vi "SEN_Loop.vi"() -> ()   [LabVIEW 2020, in "GameController_SEN.lvlib"]
uses:
  GameController_SEN.lvlib
  Shared Code/TypeDefs/Cluster_Controller Buzz.ctl
  ENUM_SEN_State.ctl
  Shared Code/TypeDefs/ENUM_Controller Buzz Select.ctl
  <vilib>/Rock Robotics/WPI/Joystick/WPI_JoystickDevRef.ctl
  <vilib>/Rock Robotics/WPI/Joystick/WPI_JoystickDeviceEnum.ctl
  ENUM_SEN_Action.ctl
  6bb8d52f-ddc5-4686-9cd9-70e339759792.vi
  bc1d27d1-f877-4a00-a1ce-faa161c31405.vi
  Utility/Global_STOP.vi
  Global_CMD_Data In.vi
  Global_SEN_Data Out.vi
panel:
  out "State":T1
  in  "Tab Control":enum32{"NONE", "Test"}(tab)
  in  "BUZZ Select":T2
  in  "BUZZ Number":dbl min=0.0 max=1.0 step=0.1 format="%.1f"
  in  "Controller BUZZ":T3
  out "Input Bool Data":bool
  out "Output DBL Data":dbl
  out "Cycle Time (S)":dbl format="%.3g"
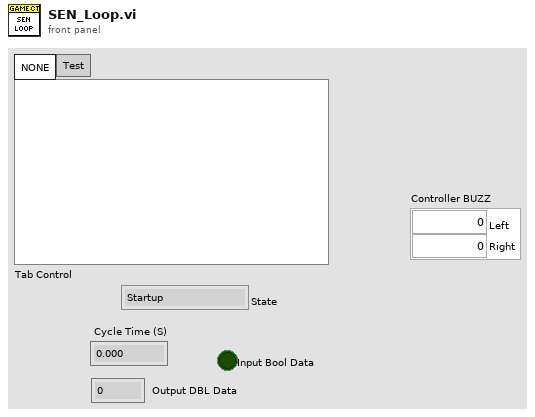
[diagram p1: front panel]
types:
  T1 = typedef "GameController_SEN.lvlib/ENUM_SEN_State.ctl" = enum16{"Startup", "Waiting BUZZ ON", "Shutdown", "Buzzing FULL Timed", "Waiting BUZZ OFF", "Buzzing Cycle Count", "Buzzing Intensity"}
  T2 = typedef "ENUM_Controller Buzz Select.ctl" = enum16{"None", "Timed Full ON", "Set Intensity", ".5 Sec Cycle Count"}
  T3 = typedef "Cluster_Controller Buzz.ctl" = cluster{"Left":dbl, "Right":dbl}
  T4 = typedef "WPI_JoystickDevRef.ctl" = cluster{"Device":T5}
  T5 = typedef "WPI_JoystickDeviceEnum.ctl" = enum16{"USB 0", "USB 1", "USB 2", "USB 3", "USB 4", "USB 5"}
  T6 = cluster{"Sensor Ref 1":T4, "Sensor Ref 0":T4, "State":T1, "Previous State":T1, "Current Time":timestamp, "Previous Time":timestamp, "Start Time":timestamp, "Target Time (ms)":u32, "Cycle Time(S)":dbl, "SEN Input":bool, "SEN Output DBL":dbl, "Read Enable":bool, "Axes 0":dbl[], "Buttons 0":bool[], "POVs 0":i16[], "Axes 1":dbl[], "Buttons 1":bool[], "POVs 1":i16[], "Controller BUZZ":T3, "BUZZ Select":T2, "BUZZ Number":dbl, "Target Number":dbl, "Count":i32, "BUZZ Target":T2}
  T7 = enum16{"Done", "First Call", "First Check", "BUZZ Match"}
  T8 = enum16{"Done", "First Call", "First Check", "BUZZ Match", "Time Expired", "Cycle Complete"}
  T9 = typedef "GameController_SEN.lvlib/ENUM_SEN_Action.ctl" = enum16{"No Action", "Reset Time", "Read Enable", "Read Disable", "SET Buzz"}
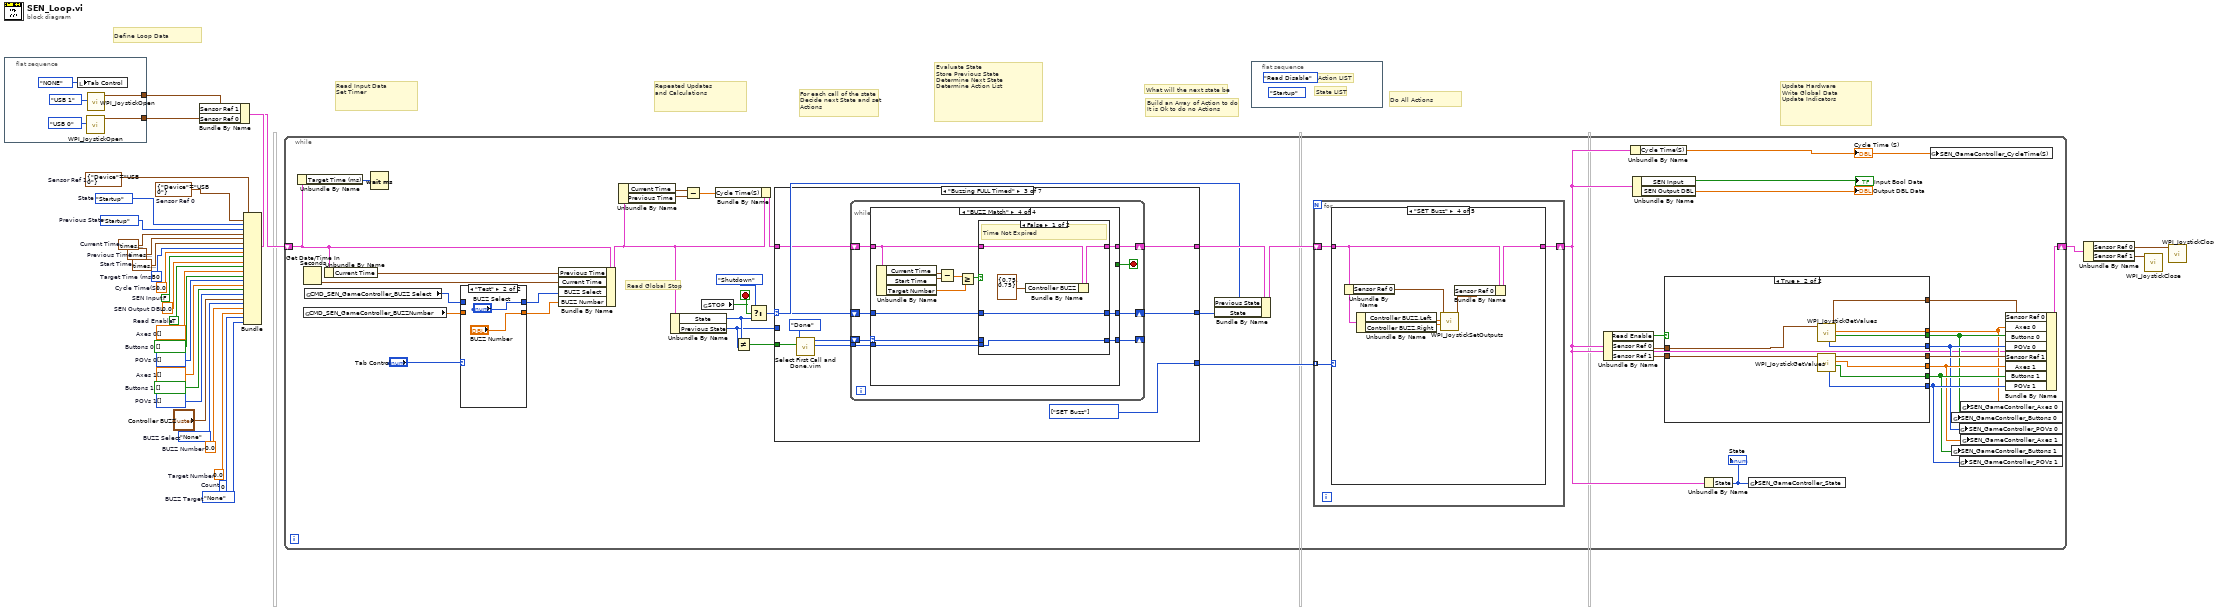
[diagram p0: block diagram]
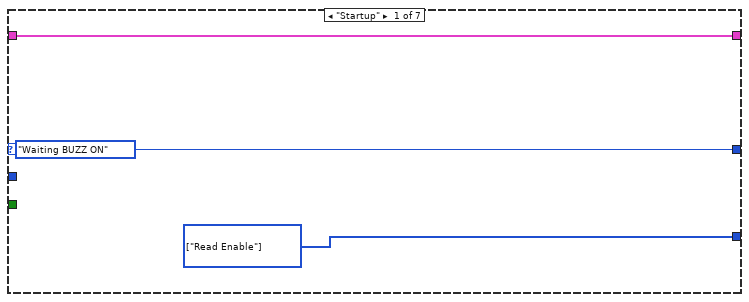
[diagram p3: hidden frame]
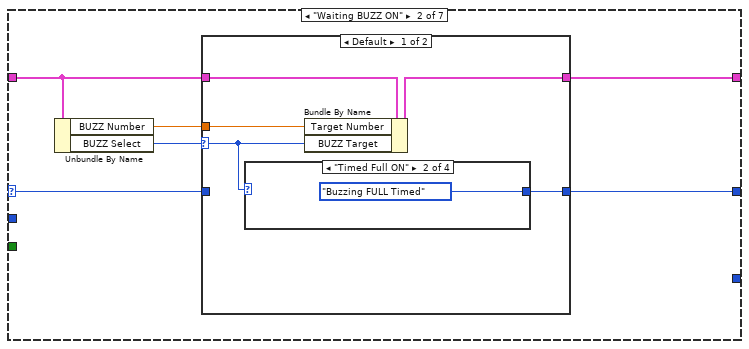
[diagram p4: hidden frame]
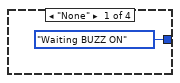
[diagram p5: hidden frame]
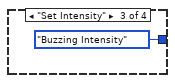
[diagram p6: hidden frame]
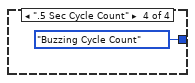
[diagram p7: hidden frame]
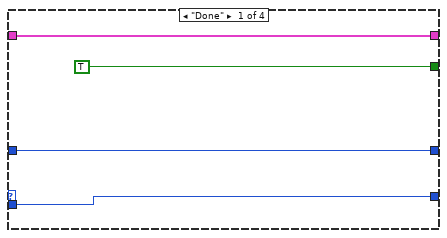
[diagram p9: hidden frame]
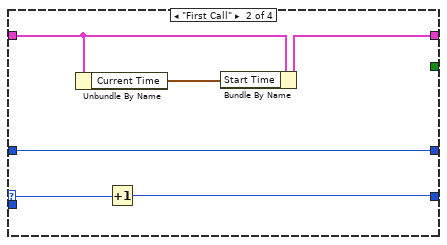
[diagram p10: hidden frame]
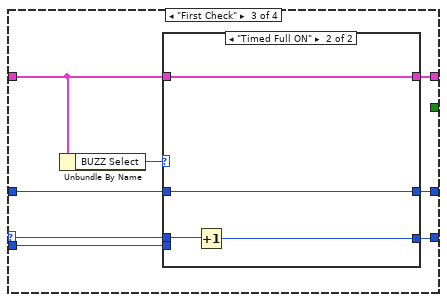
[diagram p11: hidden frame]
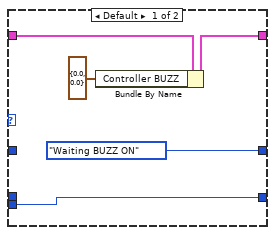
[diagram p12: hidden frame]
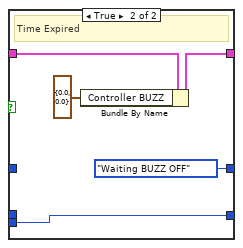
[diagram p13: hidden frame]
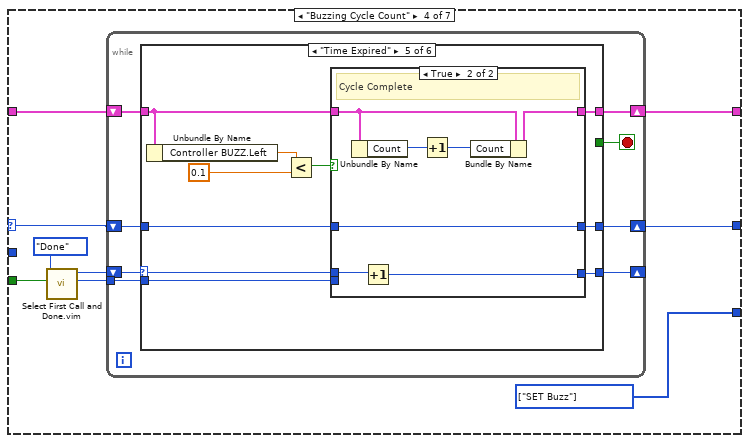
[diagram p14: hidden frame]
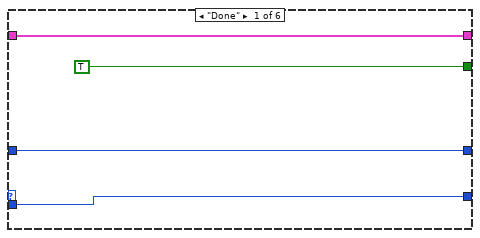
[diagram p15: hidden frame]
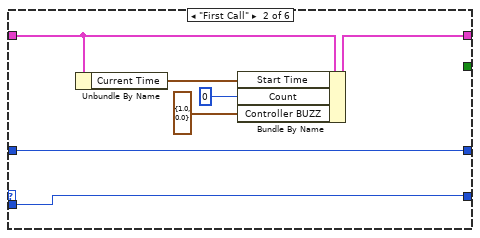
[diagram p16: hidden frame]
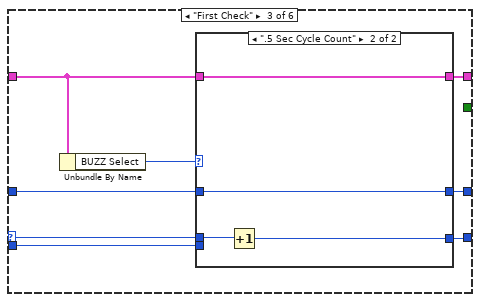
[diagram p17: hidden frame]
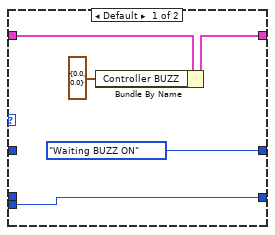
[diagram p18: hidden frame]
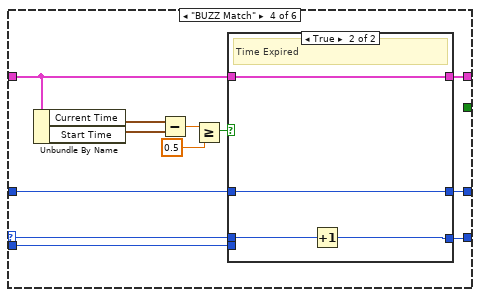
[diagram p19: hidden frame]
diagram:
  w1 = ENUM_Controller_Buzz_Select."None"  # BUZZ Target
  w2 = 0  # Count
  w3 = 0.0  # Target Number
  w4 = 0.0  # BUZZ Number
  w5 = ENUM_Controller_Buzz_Select."None"  # BUZZ Select
  w7 = T4 {"Device"=enum."USB 0"}  # Sensor Ref 0
  w8 = T4 {"Device"=enum."USB 0"}  # Sensor Ref 1
  w11 = i16[] []  # POVs 1
  w12 = bool[] []  # Buttons 1
  w13 = dbl[] []  # Axes 1
  w14 = i16[] []  # POVs 0
  w15 = bool[] []  # Buttons 0
  w16 = dbl[] []  # Axes 0
  w21 = TRUE  # Read Enable
  w23 = 0.0  # Cycle Time(S)
  w24 = ENUM_SEN_State."Startup"  # Previous State
  w25 = timestamp(0 s since 1904-01-01)  # Previous Time
  w26 = u32 50  # Target Time (ms)
  w27 = 0.0  # SEN Output DBL
  w28 = FALSE  # SEN Input
  w29 = timestamp(0 s since 1904-01-01)  # Start Time
  w30 = timestamp(0 s since 1904-01-01)  # Current Time
  w31 = ENUM_SEN_State."Startup"  # State
  # "Build an Array of Action to do\nIt is Ok to do no Actions"
  # "What will the next state be"
  # "For each call of the state\nDecide next State and set\nActions"
  # "Define Loop Data"
  # "Repeated Updates\nand Calculations"
  # "Read Input Data\nSet Timer"
  # "Evaluate State\nStore Previous State\nDetermine Next State\nDetermine Action List"
  # "Do All Actions"
  # "Update Hardware\nWrite Global Data\nUpdate Indicators"
  n1 = flat-sequence {
    tunnel: [w35] -> w18
    tunnel: [w33] -> w17
    frame #0 {
      n2 = local write "Tab Control"(enum32{"NONE", "Test"}."NONE" ("Tab Control")) -> ()
      n3 = call <vilib>:"WPI_JoystickOpen.vi"("JoystickDevice"=WPI_JoystickDeviceEnum."USB 0") -> ("JoystickDevRef"=w35:T4)  [unwired: 10 in]
      n4 = call <vilib>:"WPI_JoystickOpen.vi"("JoystickDevice"=WPI_JoystickDeviceEnum."USB 1") -> ("JoystickDevRef"=w33:T4)  [unwired: 10 in]
    }
  }
  n5 = Bundle("Sensor Ref 1"=w8, "Sensor Ref 0"=w7, "State"=w31, "Previous State"=w24, "Current Time"=w30, "Previous Time"=w25, "Start Time"=w29, "Target Time (ms)"=w26, "Cycle Time(S)"=w23, "SEN Input"=w28, "SEN Output DBL"=w27, "Read Enable"=w21, "Axes 0"=w16, "Buttons 0"=w15, "POVs 0"=w14, "Axes 1"=w13, "Buttons 1"=w12, "POVs 1"=w11, "Controller BUZZ"="Controller BUZZ", "BUZZ Select"=w5, "BUZZ Number"=w4, "Target Number"=w3, "Count"=w2, "BUZZ Target"=w1) -> (w20:T6)  [unwired: 1 in]
  n6 = Bundle By Name(cluster=w20, "Sensor Ref 1"=w17, "Sensor Ref 0"=w18) -> (w19:T6)
  n7 = while {
    shift-right: [w59] -> w22
    shift-left: w19 -> [w47]
    stop <- w73 stop-if-true
    # "Read Global Stop"
    n8 = Unbundle By Name(w47) -> ("Target Time (ms)"=w71:u32)
    n9 = global read "Global_CMD_Data In.vi" "CMD_SEN_GameController_BUZZNumber"() -> (w38:dbl)
    n10 = Get Date/Time In Seconds() -> (seconds since 1Jan1904=w77:timestamp)
    n11 = global read "Global_CMD_Data In.vi" "CMD_SEN_GameController_BUZZ Select"() -> (w40:T2)
    n12 = Unbundle By Name(w47) -> ("Current Time"=w70:timestamp)
    n13 = Wait (ms)(milliseconds to wait=w71) -> ()  [unwired: 1 out]
    n14 = case shown="\"Test\"" "Tab Control" {
      tunnel: w40 -> [w79 _]
      tunnel: w38 -> [w78 _]
      tunnel: [w79 "BUZZ Select"] -> w39
      tunnel: [w78 "BUZZ Number"] -> w37
      frame "NONE" {
      }
      frame "Test" {
      }
    }
    n15 = Bundle By Name(cluster=w47, "Previous Time"=w70, "Current Time"=w77, "BUZZ Select"=w39, "BUZZ Number"=w37) -> (w65:T6)
    n16 = Unbundle By Name(w65) -> ("Current Time"=w66:timestamp, "Previous Time"=w67:timestamp)
    n17 = Unbundle By Name(w65) -> ("State"=w44:T1, "Previous State"=w43:T1)
    n18 = Subtract(x=w66, y=w67) -> (x-y=w63:dbl)
    n19 = global read "Global_STOP.vi" "STOP"() -> (w73:bool)
    n20 = Bundle By Name(cluster=w65, "Cycle Time(S)"=w63) -> (w64:T6)
    n21 = Not Equal?(x=w44, y=w43) -> (x != y?=w42:bool)
    n22 = Select(t=ENUM_SEN_State."Shutdown" ("State"), s=w73, f=w44) -> (s? t:f=w68:T1)
    n23 = case shown="\"Buzzing FULL Timed\"" w68 {
      selector: w68 -> [_ w85 w106 w172 w278 w295 _]
      tunnel: w64 -> [w84 w88 w108 w174 w281 w297 w304]
      tunnel: [w84 w87 w107 w173 w279 w296 w304] -> w75
      tunnel: [ENUM_SEN_State."Waiting BUZZ ON" ("State") w90 w105 w171 w277 w294 ENUM_SEN_State."Shutdown" ("State")] -> w74
      tunnel: [w83 _ w102 w168 w282 _ w302] -> w62
      tunnel: w43 -> [_ _ _ _ _ _ _]
      tunnel: w42 -> [_ _ w110 w176 _ _ _]
      frame "Startup" {
        w83 = T9[] [enum."Read Enable"] items=["No Action", "Reset Time", "Read Enable", "Read Disable", "SET Buzz"] ("Actions")
      }
      frame "Waiting BUZZ ON" {
        n24 = Unbundle By Name(w88) -> ("BUZZ Number"=w86:dbl, "BUZZ Select"=w89:T2)
        n25 = case shown="Default" w89 {
          selector: w89 -> [w91 _]
          tunnel: [w95 w100] -> w90
          tunnel: w88 -> [w93 w101]
          tunnel: [w94 w101] -> w87
          tunnel: w86 -> [w92 _]
          tunnel: w85 -> [_ w100]
          frame Default {
            n26 = case shown="\"Timed Full ON\"" w91 {
              tunnel: [ENUM_SEN_State."Waiting BUZZ ON" ("State") ENUM_SEN_State."Buzzing FULL Timed" ("State") ENUM_SEN_State."Buzzing Intensity" ("State") ENUM_SEN_State."Buzzing Cycle Count" ("State")] -> w95
              frame "None" {
              }
              frame "Timed Full ON" {
              }
              frame "Set Intensity" {
              }
              frame ".5 Sec Cycle Count" {
              }
            }
            n27 = Bundle By Name(cluster=w93, "Target Number"=w92, "BUZZ Target"=w91) -> (w94:T6)
          }
          frame "None" {
          }
        }
      }
      frame "Buzzing FULL Timed" {
        w102 = T9[] [enum."SET Buzz"] items=["No Action", "Reset Time", "Read Enable", "Read Disable", "SET Buzz"] ("Actions")
        n28 = call "Select First Call and Done.vim"("First Call"=w110, "Enum 3"=T7."Done") -> ("DONE Select"=w103:T7, "First Call Select"=w104:T7)  [unwired: 8 in]
        n29 = while {
          shift-right: [w117] -> w107
          shift-left: w108 -> [w118]
          shift-right: [w114] -> w105
          shift-left: w106 -> [w115]
          shift-right: [w112] -> _
          shift-left: w104 -> [w113]
          tunnel: w103 -> [w111]
          stop <- w116 stop-if-true
          n30 = case shown="\"BUZZ Match\"" w113 {
            selector: w113 -> [_ w124 w132 w154]
            tunnel: w118 -> [w121 w126 w135 w157]
            tunnel: [w121 w127 w134 w156] -> w117
            tunnel: [TRUE _ _ _] -> w116
            tunnel: w115 -> [w120 w128 w130 w152]
            tunnel: [w120 w128 w133 w155] -> w114
            tunnel: [w119 w123 w131 w153] -> w112
            tunnel: w111 -> [w119 _ w129 w151]
            frame "Done" {
            }
            frame "First Call" {
              n31 = Unbundle By Name(w126) -> ("Current Time"=w125:timestamp)
              n32 = Increment(x=w124) -> (x+1=w123:T7)
              n33 = Bundle By Name(cluster=w126, "Start Time"=w125) -> (w127:T6)
            }
            frame "First Check" {
              n34 = Unbundle By Name(w135) -> ("BUZZ Select"=w136:T2)
              n35 = case shown="\"Timed Full ON\"" w136 {
                tunnel: w135 -> [w138 w145]
                tunnel: [w139 w145] -> w134
                tunnel: [ENUM_SEN_State."Waiting BUZZ ON" ("State") w142] -> w133
                tunnel: w132 -> [_ w144]
                tunnel: [w140 w143] -> w131
                tunnel: w130 -> [_ w142]
                tunnel: w129 -> [w140 _]
                frame Default {
                  n36 = Bundle By Name(cluster=w138, "Controller BUZZ"=T3 {"Left"=0.0, "Right"=0.0}) -> (w139:T6)
                }
                frame "Timed Full ON" {
                  n37 = Increment(x=w144) -> (x+1=w143:T7)
                }
              }
            }
            frame "BUZZ Match" {
              n38 = Unbundle By Name(w157) -> ("Current Time"=w150:timestamp, "Start Time"=w149:timestamp, "Target Number"=w147:dbl)
              n39 = Subtract(x=w150, y=w149) -> (x-y=w148:dbl)
              n40 = Greater Or Equal?(x=w148, y=w147) -> (x >= y?=w146:bool)
              n41 = case shown="False" w146 {
                tunnel: w157 -> [w159 w164]
                tunnel: [w158 w165] -> w156
                tunnel: [w161 ENUM_SEN_State."Waiting BUZZ OFF" ("State")] -> w155
                tunnel: w154 -> [_ _]
                tunnel: [w162 w167] -> w153
                tunnel: w152 -> [w161 _]
                tunnel: w151 -> [w162 w167]
                frame False {
                  # "Time Not Expired"
                  n42 = Bundle By Name(cluster=w159, "Controller BUZZ"=T3 {"Left"=0.75, "Right"=0.75}) -> (w158:T6)
                }
                frame True {
                  # "Time Expired"
                  n43 = Bundle By Name(cluster=w164, "Controller BUZZ"=T3 {"Left"=0.0, "Right"=0.0}) -> (w165:T6)
                }
              }
            }
          }
        }
      }
      frame "Buzzing Cycle Count" {
        w168 = T9[] [enum."SET Buzz"] items=["No Action", "Reset Time", "Read Enable", "Read Disable", "SET Buzz"] ("Actions")
        n44 = call "Select First Call and Done.vim"("First Call"=w176, "Enum 3"=T8."Done") -> ("DONE Select"=w169:T8, "First Call Select"=w170:T8)  [unwired: 8 in]
        n45 = while {
          shift-right: [w183] -> w173
          shift-left: w174 -> [w184]
          shift-right: [w180] -> w171
          shift-left: w172 -> [w181]
          shift-right: [w178] -> _
          shift-left: w170 -> [w179]
          tunnel: w169 -> [w177]
          stop <- w182 stop-if-true
          n46 = case shown="\"Time Expired\"" w179 {
            selector: w179 -> [_ _ w199 w221 w238 w262]
            tunnel: w184 -> [w187 w193 w202 w224 w241 w265]
            tunnel: [w187 w194 w201 w223 w240 w264] -> w183
            tunnel: [TRUE _ _ _ _ _] -> w182
            tunnel: w181 -> [w186 w195 w197 w219 w236 w260]
            tunnel: [w186 w195 w200 w222 w239 w263] -> w180
            tunnel: [w185 w189 w198 w220 w237 w261] -> w178
            tunnel: w177 -> [w185 w189 w196 w218 w235 w259]
            frame "Done" {
            }
            frame "First Call" {
              n47 = Unbundle By Name(w193) -> ("Current Time"=w192:timestamp)
              n48 = Bundle By Name(cluster=w193, "Start Time"=w192, "Count"=0, "Controller BUZZ"=T3 {"Left"=1.0, "Right"=0.0}) -> (w194:T6)
            }
            frame "First Check" {
              n49 = Unbundle By Name(w202) -> ("BUZZ Select"=w203:T2)
              n50 = case shown="\".5 Sec Cycle Count\"" w203 {
                tunnel: w202 -> [w205 w212]
                tunnel: [w206 w212] -> w201
                tunnel: [ENUM_SEN_State."Waiting BUZZ ON" ("State") w209] -> w200
                tunnel: w199 -> [_ w211]
                tunnel: [w207 w210] -> w198
                tunnel: w197 -> [_ w209]
                tunnel: w196 -> [w207 _]
                frame Default {
                  n51 = Bundle By Name(cluster=w205, "Controller BUZZ"=T3 {"Left"=0.0, "Right"=0.0}) -> (w206:T6)
                }
                frame ".5 Sec Cycle Count" {
                  n52 = Increment(x=w211) -> (x+1=w210:T8)
                }
              }
            }
            frame "BUZZ Match" {
              n53 = Unbundle By Name(w224) -> ("Current Time"=w217:timestamp, "Start Time"=w216:timestamp)
              n54 = Subtract(x=w217, y=w216) -> (x-y=w215:dbl)
              n55 = Greater Or Equal?(x=w215, y=0.5) -> (x >= y?=w214:bool)
              n56 = case shown="True" w214 {
                tunnel: w224 -> [w225 w231]
                tunnel: [w225 w231] -> w223
                tunnel: [w226 w230] -> w222
                tunnel: w221 -> [_ w229]
                tunnel: [w227 w228] -> w220
                tunnel: w219 -> [w226 w230]
                tunnel: w218 -> [w227 _]
                frame False {
                  # "Time Not Expired"
                }
                frame True {
                  # "Time Expired"
                  n57 = Increment(x=w229) -> (x+1=w228:T8)
                }
              }
            }
            frame "Time Expired" {
              n58 = Unbundle By Name(w241) -> ("Controller BUZZ.Left"=w233:dbl)
              n59 = Less?(x=w233, y=0.1) -> (x < y?=w234:bool)
              n60 = case shown="True" w234 {
                tunnel: w241 -> [w244 w250]
                tunnel: [w245 w251] -> w240
                tunnel: [w246 w254] -> w239
                tunnel: w238 -> [_ w253]
                tunnel: [w247 w252] -> w237
                tunnel: w236 -> [w246 w254]
                tunnel: w235 -> [w247 _]
                frame False {
                  # "First half of cycle"
                  n61 = Unbundle By Name(w244) -> ("Current Time"=w243:timestamp)
                  n62 = Bundle By Name(cluster=w244, "Start Time"=w243, "Controller BUZZ"=T3 {"Left"=0.0, "Right"=1.0}) -> (w245:T6)
                }
                frame True {
                  # "Cycle Complete"
                  n63 = Unbundle By Name(w250) -> ("Count"=w249:i32)
                  n64 = Increment(x=w253) -> (x+1=w252:T8)
                  n65 = Increment(x=w249) -> (x+1=w248:i32)
                  n66 = Bundle By Name(cluster=w250, "Count"=w248) -> (w251:T6)
                }
              }
            }
            frame "Cycle Complete" {
              n67 = Unbundle By Name(w265) -> ("Count"=w256:i32, "Target Number"=w255:dbl)
              n68 = To Long Integer(number=w255) -> (32bit integer=w257:i32)
              n69 = Greater Or Equal?(x=w256, y=w257) -> (x >= y?=w258:bool)
              n70 = case shown="False" w258 {
                tunnel: w265 -> [w268 w273]
                tunnel: [w269 w274] -> w264
                tunnel: [w270 ENUM_SEN_State."Waiting BUZZ OFF" ("State")] -> w263
                tunnel: w262 -> [_ _]
                tunnel: [w271 w276] -> w261
                tunnel: w260 -> [w270 _]
                tunnel: w259 -> [w271 w276]
                frame False {
                  # "Count Not complete"
                  n71 = Unbundle By Name(w268) -> ("Current Time"=w267:timestamp)
                  n72 = Bundle By Name(cluster=w268, "Start Time"=w267, "Controller BUZZ"=T3 {"Left"=1.0, "Right"=0.0}) -> (w269:T6)
                }
                frame True {
                  # "Count Complete"
                  n73 = Bundle By Name(cluster=w273, "Controller BUZZ"=T3 {"Left"=0.0, "Right"=0.0}) -> (w274:T6)
                }
              }
            }
          }
        }
      }
      frame "Buzzing Intensity" {
        w282 = T9[] [enum."SET Buzz"] items=["No Action", "Reset Time", "Read Enable", "Read Disable", "SET Buzz"] ("Actions")
        n74 = Unbundle By Name(w281) -> ("BUZZ Select"=w280:T2)
        n75 = case shown="Default" w280 {
          tunnel: w281 -> [w284 w288]
          tunnel: [w285 w289] -> w279
          tunnel: w278 -> [_ w290]
          tunnel: [ENUM_SEN_State."Waiting BUZZ ON" ("State") w290] -> w277
          frame Default {
            n76 = Bundle By Name(cluster=w284, "Controller BUZZ"=T3 {"Left"=0.0, "Right"=0.0}) -> (w285:T6)
          }
          frame "Set Intensity" {
            n77 = Unbundle By Name(w288) -> ("BUZZ Number"=w287:dbl)
            n78 = Bundle By Name(cluster=w288, "Controller BUZZ.Left"=w287, "Controller BUZZ.Right"=w287) -> (w289:T6)
          }
        }
      }
      frame "Waiting BUZZ OFF" {
        n79 = Unbundle By Name(w297) -> ("BUZZ Target"=w293:T2, "BUZZ Select"=w292:T2)
        n80 = Not Equal?(x=w293, y=w292) -> (x != y?=w291:bool)
        n81 = case shown="False" w291 {
          tunnel: w297 -> [w298 w300]
          tunnel: [w298 w300] -> w296
          tunnel: w295 -> [w299 _]
          tunnel: [w299 ENUM_SEN_State."Waiting BUZZ ON" ("State")] -> w294
          frame False {
            # "Same Target"
          }
          frame True {
            # "New Target"
          }
        }
      }
      frame "Shutdown" {
        w302 = T9[] [enum."Read Disable"] items=["No Action", "Reset Time", "Read Enable", "Read Disable", "SET Buzz"] ("Actions")
      }
    }
    n82 = Bundle By Name(cluster=w75, "Previous State"=w68, "State"=w74) -> (w76:T6)
    n83 = for {
      tunnel: w62 -> [w319] mode=indexing
      shift-right: [w318] -> w46
      shift-left: w76 -> [w317]
      n84 = case shown="\"SET Buzz\"" w319 {
        tunnel: w317 -> [w320 w323 w326 w327 w335]
        tunnel: [w320 w322 w325 w329 w334] -> w318
        frame "No Action" {
        }
        frame "Reset Time" {
          # "Reset timer by taking the current time\nand making it the start time\n\nLater when the current time is \nsubtracted from the start time\nyou will get the elapsed time in \nseconds"
          n85 = Unbundle By Name(w323) -> ("Current Time"=w321:timestamp)
          n86 = Bundle By Name(cluster=w323, "Start Time"=w321) -> (w322:T6)
        }
        frame "Read Enable" {
          n87 = Bundle By Name(cluster=w326, "Read Enable"=TRUE) -> (w325:T6)
        }
        frame "SET Buzz" {
          n88 = Unbundle By Name(w327) -> ("Sensor Ref 0"=w330:T4)
          n89 = Unbundle By Name(w327) -> ("Controller BUZZ.Left"=w332:dbl, "Controller BUZZ.Right"=w331:dbl)
          n90 = call <vilib>:"WPI_JoystickSetOutputs.vi"("Right Rumble"=w331, "Left Rumble"=w332, "JoystickDevRef"=w330) -> ("JoystickDevRef"=w328:T4)  [unwired: 7 in, 1 out]
          n91 = Bundle By Name(cluster=w327, "Sensor Ref 0"=w328) -> (w329:T6)
        }
        frame "Read Disable" {
          n92 = Bundle By Name(cluster=w335, "Read Enable"=FALSE) -> (w334:T6)
        }
      }
    }
    n93 = Unbundle By Name(w46) -> ("Read Enable"=w57:bool, "Sensor Ref 0"=w60:T4, "Sensor Ref 1"=w56:T4)
    n94 = Unbundle By Name(w46) -> ("Cycle Time(S)"=w58:dbl)
    "Cycle Time (S)" <- w58
    n95 = Unbundle By Name(w46) -> ("SEN Input"=→"Input Bool Data":bool, "SEN Output DBL"=→"Output DBL Data":dbl)
    n96 = case shown="True" w57 {
      tunnel: w60 -> [w306 w308]
      tunnel: [w305 w316] -> w54
      tunnel: w56 -> [w305 w309]
      tunnel: [w306 w307] -> w55
      tunnel: [_ w315] -> w48
      tunnel: [_ w314] -> w49
      tunnel: [_ w313] -> w50
      tunnel: [_ w312] -> w51
      tunnel: [_ w311] -> w52
      tunnel: [_ w310] -> w53
      frame False {
      }
      frame True {
        n97 = call <vilib>:"WPI_JoystickGetValues.vi"("JoystickDevRef"=w308) -> ("Buttons"=w314:bool[], "Axes"=w315:dbl[], "JoystickDevRef"=w307:T4, "POVs"=w313:i16[])  [unwired: 6 in, 1 out]
        n98 = call <vilib>:"WPI_JoystickGetValues.vi"("JoystickDevRef"=w309) -> ("Buttons"=w311:bool[], "Axes"=w312:dbl[], "JoystickDevRef"=w316:T4, "POVs"=w310:i16[])  [unwired: 6 in, 1 out]
      }
    }
    n99 = Unbundle By Name(w46) -> ("State"=w45:T1)
    "State" <- w45
    n100 = global write "Global_SEN_Data Out.vi" "SEN_GameController_State"(w45) -> ()
    n101 = global write "Global_SEN_Data Out.vi" "SEN_GameController_CycleTime(S)"(w58) -> ()
    n102 = global write "Global_SEN_Data Out.vi" "SEN_GameController_Buttons 0"(w49) -> ()
    n103 = global write "Global_SEN_Data Out.vi" "SEN_GameController_Buttons 1"(w52) -> ()
    n104 = global write "Global_SEN_Data Out.vi" "SEN_GameController_POVs 0"(w50) -> ()
    n105 = global write "Global_SEN_Data Out.vi" "SEN_GameController_POVs 1"(w53) -> ()
    n106 = global write "Global_SEN_Data Out.vi" "SEN_GameController_Axes 0"(w48) -> ()
    n107 = global write "Global_SEN_Data Out.vi" "SEN_GameController_Axes 1"(w51) -> ()
    n108 = Bundle By Name(cluster=w46, "Sensor Ref 0"=w55, "Axes 0"=w48, "Buttons 0"=w49, "POVs 0"=w50, "Sensor Ref 1"=w54, "Axes 1"=w51, "Buttons 1"=w52, "POVs 1"=w53) -> (w59:T6)
  }
  n109 = flat-sequence {
    frame #0 {
      (unwired) ENUM_SEN_State."Startup" ("State")
      (unwired) ENUM_SEN_Action."Read Disable" ("Action")
      # "State LIST"
      # "Action LIST"
    }
  }
  n110 = Unbundle By Name(w22) -> ("Sensor Ref 0"=w10:T4, "Sensor Ref 1"=w9:T4)
  n111 = call <vilib>:"WPI_JoystickClose.vi"("JoystickDevRef"=w9) -> ()  [unwired: 11 in]
  n112 = call <vilib>:"WPI_JoystickClose.vi"("JoystickDevRef"=w10) -> ()  [unwired: 11 in]
